vi "LVH5 Write Attributes_AdaptToInputs.vi"(3 "Term Types":T1[](array[typedef]), 4 "XRef":refnum<vi>, 5 "State In":T4) -> (0 "Reply":string[](array[string]), 2 "State Out":T4)   [LabVIEW 2017, in "LVH5 Write Attributes.xnode"]
uses:
  <vilib>/UPVI/lvhdf5/attribute.llb/LVH5 Write Attributes.xnode
  <vilib>/UPVI/lvhdf5/attribute.llb/LVH5 Write Attributes/LVH5 Write Attributes_State.ctl
  <vilib>/UPVI/lvhdf5/xnodehelpers/TermsPlus.ctl
  <vilib>/XNodeSupport/XNodeTerm3.ctl
  <vilib>/XNodeSupport/XNodeString.ctl
  <vilib>/XNodeSupport/XNodeVariant.ctl
  <vilib>/XNodeSupport/XNodeRect32.ctl
  <vilib>/XNodeSupport/XNodeInt.ctl
  <vilib>/XNodeSupport/XNodeBool.ctl
  <vilib>/XNodeSupport/XNodeTermDirection.ctl
  <vilib>/UPVI/lvhdf5/xnodehelpers/TermBehavior.ctl
  <vilib>/XNodeSupport/XNodeError3Array.ctl
  <vilib>/XNodeSupport/XNodeError3.ctl
  <vilib>/XNodeSupport/XNodeTermTypeIDPair.ctl
  <vilib>/XNodeSupport/XNodeType.ctl
  <vilib>/XNodeSupport/NI_XNodeSupport.lvlib
panel:
  # "LVHDF5 Toolkit\nCopyright (c) 2005-2013 by Jason D. Sommerville\nCopyright (c) 2014 by UPVI, LLC.\n\nThis use and distribution of this file is governed by the terms found in \nLICENSE.txt distributed with this toolkit and installed at\n <user.lib>\\_lvhdf5\\LICENSE.txt"
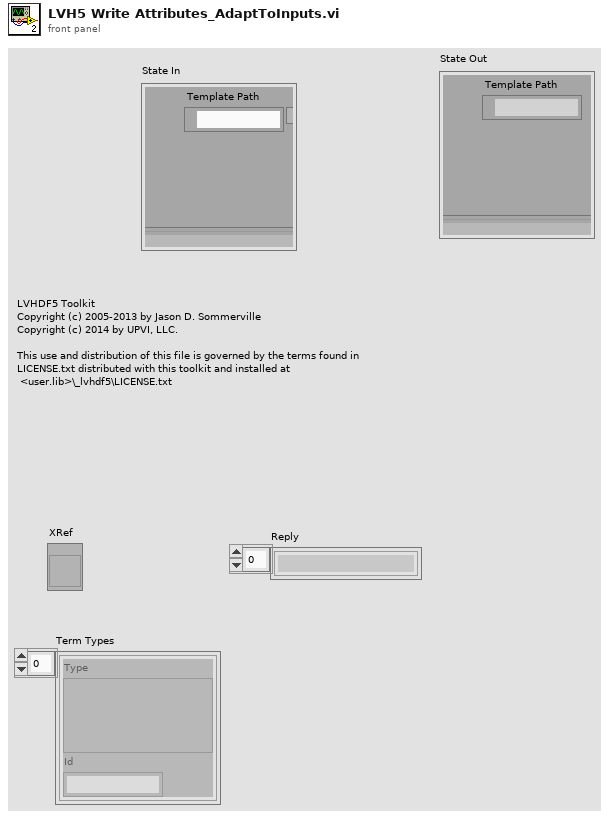
[diagram p1: front panel]
types:
  T1 = typedef "NI_XNodeSupport.lvlib/XNodeTermTypeIDPair.ctl" = cluster{"Type":T2, "Id":T3}
  T2 = typedef "NI_XNodeSupport.lvlib/XNodeType.ctl" = variant
  T3 = typedef "NI_XNodeSupport.lvlib/XNodeString.ctl" = string
  T4 = typedef "LVH5 Write Attributes.xnode/LVH5 Write Attributes_State.ctl" = cluster{"Template Path":path, "Template Ref":refnum<vi>, "Terms":T5[], "Display Name":string, "Image":picture, "Errors":T13, "Generated?":bool, "Mode":enum16{"<Invalid>", "Single", "Multiple", "Cluster"}, "Mode Images":picture[]}
  T5 = typedef "TermsPlus.ctl" = cluster{"Term 3":T6, "Default Type":variant, "Behavior":T12, "Behavior Arg":string, "WiredResponse":bool, "Wired":enum16{"Unknown", "Unwired", "Wired"}}
  T6 = typedef "NI_XNodeSupport.lvlib/XNodeTerm3.ctl" = cluster{"Name":T3, "Id":T3, "Type":T7, "Bounds":T8, "Input?":T10, "Required?":T10, "Recommended?":T10, "Adaptive?":T10, "Hidden?":T10, "Direction":T11, "Break Wire?":T10}
  T7 = typedef "NI_XNodeSupport.lvlib/XNodeVariant.ctl" = variant
  T8 = typedef "NI_XNodeSupport.lvlib/XNodeRect32.ctl" = cluster{"Left":T9, "Top":T9, "Right":T9, "Bottom":T9}
  T9 = typedef "NI_XNodeSupport.lvlib/XNodeInt.ctl" = i32
  T10 = typedef "NI_XNodeSupport.lvlib/XNodeBool.ctl" = bool
  T11 = typedef "NI_XNodeSupport.lvlib/XNodeTermDirection.ctl" = enum32{"Auto", "Up", "Down", "Left", "Right", "Center"}
  T12 = typedef "TermBehavior.ctl" = enum16{"Normal", "Anything", "LVType", "Path or Ref", "Attr Name", "Attr Poly", "Elt Poly", "Dset Poly", "WDT Poly"}
  T13 = typedef "NI_XNodeSupport.lvlib/XNodeError3Array.ctl" = T14[]
  T14 = typedef "NI_XNodeSupport.lvlib/XNodeError3.ctl" = cluster{"Error":T3, "Details":T3, "Help File":T3, "Help Topic":T3}
  T15 = enum16{"<Invalid>", "Single", "Multiple", "Cluster"}
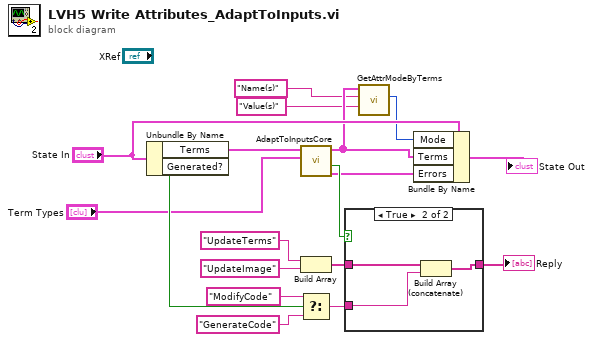
[diagram p0: block diagram]
diagram:
  n1 = Unbundle By Name("State In") -> ("Terms"=w11:T5[], "Generated?"=w12:bool)
  n2 = call <vilib>:"AdaptToInputsCore.vi"("Wired Terms"="Term Types", "Template Terms"=w11) -> ("Errors out"=w9:T14[], "Terms Modified?"=w10:bool, "Terms Out"=w4:T5[])  [unwired: 7 in]
  n3 = Build Array("UpdateTerms" ("String"), "UpdateImage" ("element")) -> (w17:string[])
  n4 = Select(t="ModifyCode", s=w12, f="GenerateCode") -> (s? t:f=w14:string)
  n5 = case shown="True" w10 {
    tunnel: w17 -> [w19 w22]
    tunnel: [w19 w21] -> w5
    tunnel: w14 -> [_ w20]
    frame False {
    }
    frame True {
      n6 = Build Array (concatenate)(w22, w20) -> (w21:string[])
    }
  }
  "Reply" <- w5
  n7 = call <vilib>:"GetAttrModeByTerms.vi"("Attr Type Term Id"="Value(s)", "Attr Name Term Id"="Name(s)", "Template Terms"=w4) -> ("Mode"=w1:T15)  [unwired: 8 in]
  n8 = Bundle By Name(cluster="State In", "Mode"=w1, "Terms"=w4, "Errors"=w9) -> (→"State Out":T4)
